vi "CleanUp.vi"(8 "error in (no error)":errorcluster, 11 "humiditySensor in":refnum<class "humiditySensor.lvclass">) -> (0 "error out":errorcluster, 3 "humiditySensor out":refnum<class "humiditySensor.lvclass">)   [LabVIEW 2020, in "RPI.SenseHat.Sensors.lvlib" / "humiditySensor.lvclass"]
uses:
  humiditySensor.lvclass
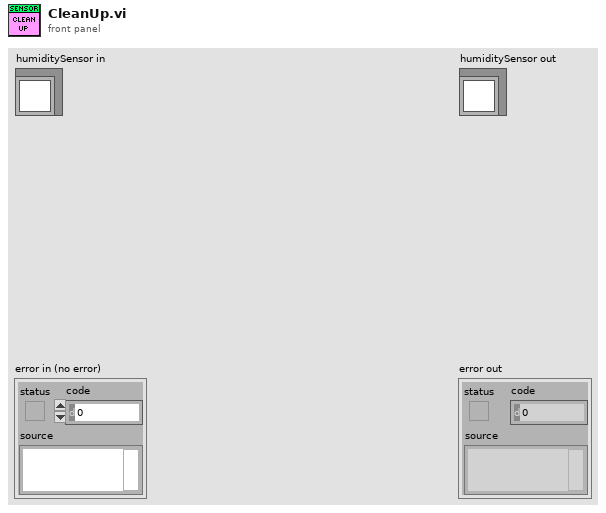
[diagram p1: front panel]
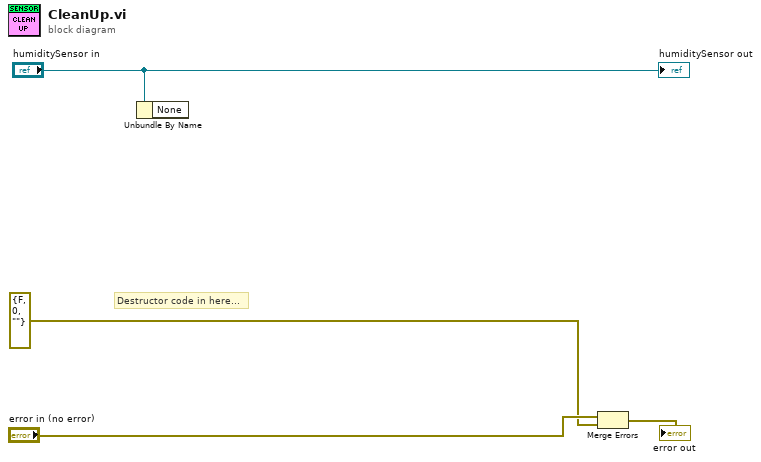
[diagram p0: block diagram]
diagram:
  # "Destructor code in here..."
  n1 = Unbundle By Name("humiditySensor in") -> ()  [unwired: 1 out]
  n2 = Merge Errors("error in (no error)", errorcluster {"status"=FALSE, "code"=0, "source"=""} ("error in (no error)")) -> (→"error out":errorcluster)
  "humiditySensor out" <- "humiditySensor in"
